vi "List Instances.vi"(8 "error in":errorcluster) -> (0 "error out":errorcluster, 2 "First Module ID":i32, 3 "Module IDs":i32[](array[numeric]), 4 "First?":bool[](array[boolean]), 5 "Instances Names":string[](array[string]))   [LabVIEW 2024, in "Cloneable Subpanel.lvlib" / "Clone Registration.lvlib"]
doc: "Retrieve information on all cloneable modules stored in the registry.\n_____\nBased on DQMH Dev Tools: Project Template 7.1.0.1499."
uses:
  Clone Registration.lvlib
  Action--enum.ctl
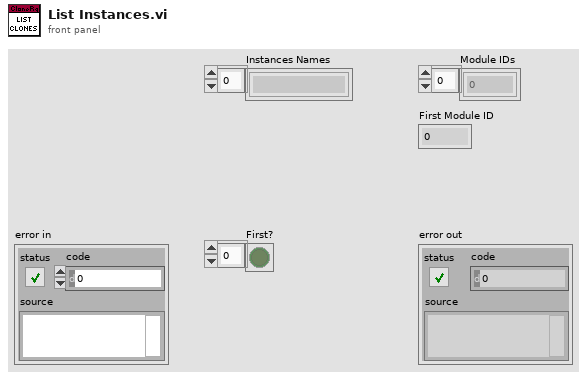
[diagram p1: front panel]
types:
  T1 = typedef "Cloneable Subpanel.lvlib/Clone Registration.lvlib/Action--enum.ctl" = enum16{"Init", "Add Instance", "Remove Instance", "List Instances", "Is First?"}
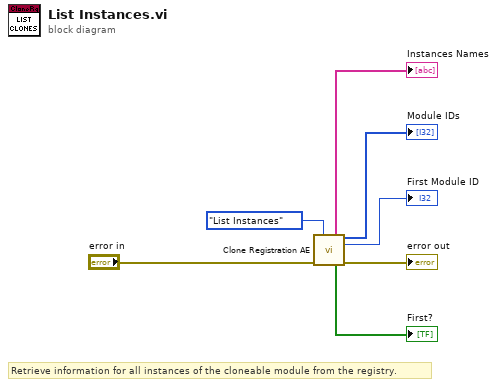
[diagram p0: block diagram]
diagram:
  # "Retrieve information for all instances of the cloneable module from the registry."
  n1 = call "Clone Registration AE.vi"("Action"=Action--enum."List Instances", "error in"="error in") -> ("Instances Names"=→"Instances Names":string[], "Module IDs"=→"Module IDs":i32[], "First Module ID"=→"First Module ID":i32, "First? (all)"=→"First?":bool[], "error out"=→"error out":errorcluster)  [unwired: 5 in, 4 out]
